vi "TSM Relay Control Session Single Action.vi"(0 "TSM Relay in":T1={"TSM context"=refnum, "Pin Query Context"=refnum, "TSM Site Numbers"=[], "SSC Relay"=[], "Unfiltered Pins"=[], "Filtered Pins"=[], "Filtered Pins Info"={"Unfiltered Pins Count"=3, "Locations"=[], "Lengths"=[]}}, 5 "Relay Action":T6=21 items=["Open Relay"=20, "Close Relay"=21], 7 "Settling Time (s)":dbl, 11 "error in":errorcluster) -> (4 "TSM Relay out":T1={"TSM context"=refnum, "Pin Query Context"=refnum, "TSM Site Numbers"=[], "SSC Relay"=[], "Unfiltered Pins"=[], "Filtered Pins"=[], "Filtered Pins Info"={"Unfiltered Pins Count"=3, "Locations"=[], "Lengths"=[]}}, 8 "Completed Relay Operations":T5[](array[typedef]) {"Desired State" items=["Open Relay"=20, "Close Relay"=21]}, 15 "error out":errorcluster)   [LabVIEW 2019]
doc: "Performs the specified relay action on all Relays configured in the TSM Relay session. The function will then wait a specified amount of time if the Settling Time (s) input is wired."
uses:
  <instrlib>/niSwitch/niSwitch.llb/niSwitch Relay Action.ctl
  SubVIs/TSM SSC Relay.ctl
  <vilib>/NI_TestStand_SemiconductorModule/NI_TestStand_Semiconductor_Module.lvlibp/PinMap/PinQueryContext/MultiplePinMultipleSessionQueryContext/MultiplePinMultipleSessionQueryContext.lvclass
  <vilib>/NI_TestStand_SemiconductorModule/NI_TestStand_Semiconductor_Module.lvlibp/PinMap/General/SemiconductorModuleContext.ctl
  SSC/SSC Relay.ctl
  SubVIs/TSM Filtered Pins Info.ctl
  SubVIs/TSM Relay Completed Operations.ctl
  SSC/SSC Relay Control/SSC Relay Control Single Action.vi
  SSC/SSC Relay Control Core.vi
  SSC/Single SSC Relay NI-Switch Control.vi
  SSC/Single SSC Relay Fill Additional Error info.vi
  SSC/SSC Relay Expand Action Array to All Sessions.vi
  <vilib>/Utility/error.llb/Error Cluster From Error Code.vi
  <instrlib>/niSwitch/niSwitch.llb/niSwitch Get Relay Position.vi
  <instrlib>/niSwitch/niSwitch.llb/niSwitch Relay Control.vi
  <vilib>/Utility/High Resolution Polling Wait.vi
  <vilib>/NI_TestStand_SemiconductorModule/NI_TestStand_Semiconductor_Module.lvlibp
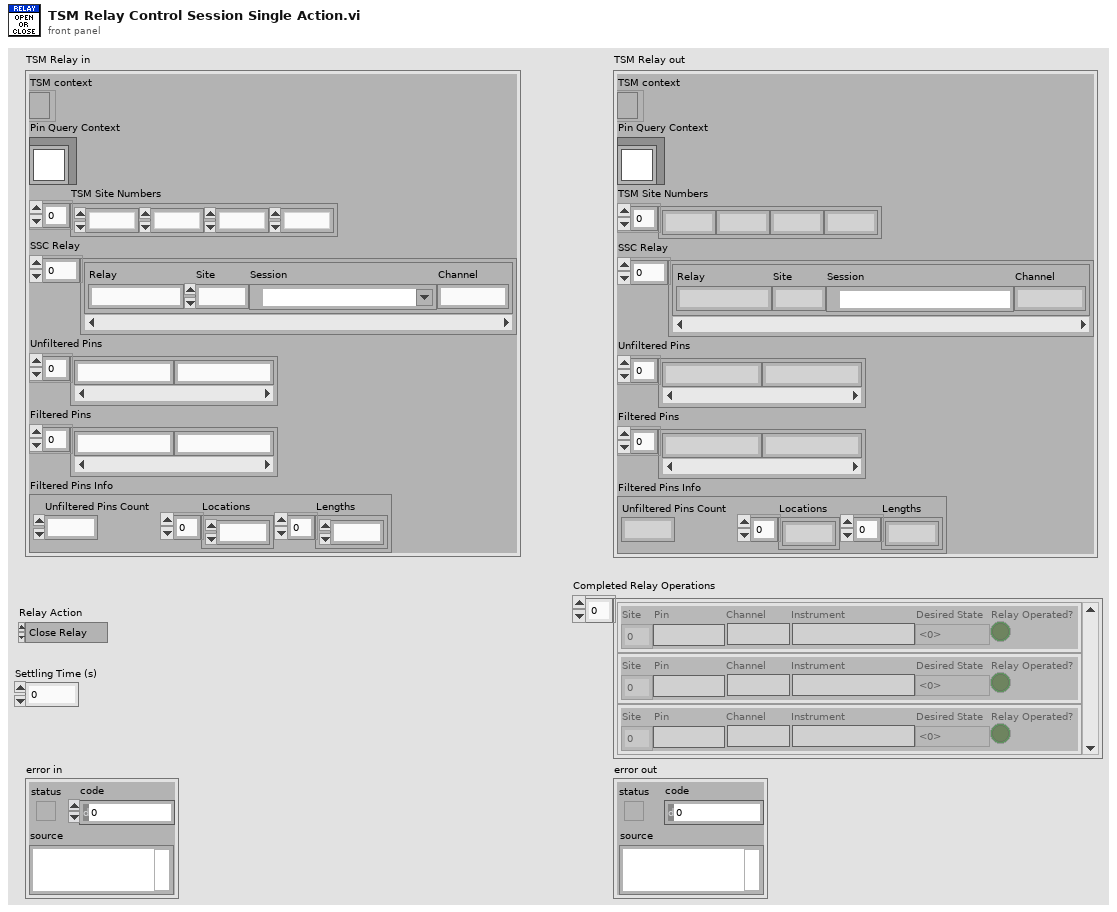
[diagram p1: front panel]
types:
  T1 = typedef "TSM SSC Relay.ctl" = cluster{"TSM context":T2, "Pin Query Context":refnum<class "MultiplePinMultipleSessionQueryContext.lvclass">, "TSM Site Numbers":i32[], "SSC Relay":T3[], "Unfiltered Pins":string[], "Filtered Pins":string[], "Filtered Pins Info":T4}
  T2 = typedef "NI_TestStand_Semiconductor_Module.lvlibp/SemiconductorModuleContext.ctl" = refnum<k7>
  T3 = typedef "SSC Relay.ctl" = cluster{"Relay":string, "Site":i32, "Session":refnum<k15>, "Channel":string}
  T4 = typedef "TSM Filtered Pins Info.ctl" = cluster{"Unfiltered Pins Count":i32, "Locations":i32[], "Lengths":i32[]}
  T5 = typedef "TSM Relay Completed Operations.ctl" = cluster{"Site":i32, "Pin":string, "Channel":string, "Instrument":string, "Desired State":T6, "Relay Operated?":bool}
  T6 = typedef "niSwitch Relay Action.ctl" = i32
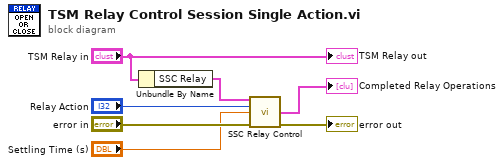
[diagram p0: block diagram]
diagram:
  n1 = Unbundle By Name("TSM Relay in") -> ("SSC Relay"=w1:T3[])
  n2 = call-poly "SSC Relay Control.vi"("SSC Relay in"=w1, "Relay Action"="Relay Action", "Settling Time (s)"="Settling Time (s)", "error in"="error in") -> ("Completed Relay Operations"=→"Completed Relay Operations":T5[], "error out"=→"error out":errorcluster)  [unwired: 9 in, 1 out]
  "TSM Relay out" <- "TSM Relay in"
